vi "Convert Spreadsheet Text to Table.vi"(1 "NumCols":i32=19, 2 "Text In":string="Date: \t8/30/2005\r\nTime: \t7:47 PM\r\nFilename: \tC:\\ER2005\\Data\\Cell 6A Data.dat\r\nProject: \tCell 6A Project\r\nSample ID: \tSample 6A\r\nRock Type: \tRock 6A\r\nFluid Pair: \tmud and guts\r\nRW: \t2.000\r\nRW Temp: \t22.0\r\nFrequency: \t1000\r\nAmplitude: \t1\r\nDAQ Period (mins): \t15\r\nLength: \t10.0000\r\nDiameter: \t5.0000\r\nPorosity: \t33.00\r\nPermeability: \t6.00\r\nElect Spacing: \t5.00\r\n\r\n Point\t Point\t Point\tEl-Time\t ER 1-2\t ER 1-3\t ER 1-4\t ER 2-3\t F 2-3\t Temp-A\t Temp-B\t  NOP\t   Pc\t P-Vol\t  C14\t  C23\r\n  Flag\t  Date\t  Time\t(Hours)\t(ohm-m)\t(ohm-m)\t(ohm-m)\t(ohm-m)\t  ()  \t(deg-C)\t(deg-C)\t (psig)\t (psig)\t  (ml)\t  (pf)\t  (pf)\r\n-------\t-------\t-------\t-------\t-------\t-------\t-------\t-------\t-------\t-------\t-------\t-------\t-------\t-------\t-------\t-------\r\n       \t8/30/05\t 19:47\t   0.00\t 78.495\t 26.215\t 19.742\t  0.075\t    0.8\t  944.1\t  944.0\t    -13\t 113.87\t   0.00\t   9170\t-1836892\r\n   V   \t8/30/05\t 19:55\t   0.14\t 78.256\t 26.179\t 19.715\t  0.178\t    2.0\t  944.0\t  943.9\t      3\t 114.10\t   1.00\t   8175\t-15739120\r\n       \t8/30/05\t 20:01\t   0.23\t 79.415\t 26.786\t 20.250\t  0.472\t    5.2\t  944.0\t  943.9\t      9\t 114.19\t   1.00\t   8342\t 859846\r\n       \t8/30/05\t 20:15\t   0.48\t 79.679\t 26.786\t 20.200\t  0.348\t    3.9\t  944.2\t  944.1\t     -0\t 114.17\t   1.00\t   7967\t-1701240\r\n       \t8/30/05\t 20:30\t   0.73\t 78.752\t 26.296\t 19.774\t  0.073\t    0.8\t  944.7\t  944.6\t      0\t 114.30\t   1.00\t  13499\t-15913632\r\n       \t8/30/05\t 20:45\t   0.98\t 78.717\t 26.274\t 19.757\t  0.053\t    0.6\t  945.4\t  945.3\t     -1\t 114.40\t   1.00\t   7499\t-4510277\r\n       \t8/30/05\t 21:00\t   1.23\t 78.693\t 26.265\t 19.739\t  0.059\t    0.7\t  946.0\t  946.0\t     -4\t 114.44\t   1.00\t   6891\t-35104476\r\n       \t8/30/05\t 21:45\t   1.98\t 78.646\t 26.296\t 19.787\t  0.122\t    1.4\t  946.9\t  946.8\t     -1\t 114.63\t   1.00\t  10271\t3895880\r\n       \t8/30/05\t 22:00\t   2.23\t 78.773\t 26.317\t 19.792\t  0.117\t    1.3\t  947.0\t  946.9\t      2\t 114.68\t   1.00\t   7326\t-26200800\r\n       \t8/30/05\t 22:15\t   2.48\t 78.537\t 26.199\t 19.678\t  0.078\t    0.9\t  947.1\t  947.0\t     -4\t 114.60\t   1.00\t   6067\t-94763630\r\n       \t8/30/05\t 22:30\t   2.73\t 78.642\t 26.240\t 19.708\t  0.090\t    1.0\t  947.1\t  947.0\t      1\t 114.65\t   1.00\t   9512\t-69234673\r\n       \t8/30/05\t 22:45\t   2.98\t 78.652\t 26.227\t 19.714\t  0.014\t    0.2\t  947.1\t  947.0\t     -4\t 114.62\t   1.00\t  14912\t53204022\r\n       \t8/30/05\t 23:00\t   3.23\t 78.582\t 26.218\t 19.703\t  0.041\t    0.5\t  947.1\t  947.0\t     -2\t 114.61\t   1.00\t  11239\t72768719\r\n       \t8/30/05\t 23:30\t   3.73\t 78.459\t 26.247\t 19.741\t  0.167\t    1.9\t  947.1\t  947.0\t    -15\t 114.40\t   1.00\t   8726\t18480066\r\n       \t8/30/05\t 23:45\t   3.98\t 78.835\t 26.447\t 20.018\t  0.275\t    3.1\t  947.0\t  946.9\t     -2\t 114.54\t   1.00\t  14136\t-4576243\r\n       \t8/31/05\t 00:00\t   4.23\t 78.781\t 26.326\t 19.809\t  0.106\t    1.2\t  946.9\t  946.8\t      1\t 114.55\t   1.00\t   8822\t-11848964\r\n       \t8/31/05\t 00:15\t   4.48\t 78.641\t 26.836\t 20.722\t  0.977\t   10.9\t  947.0\t  946.8\t     -7\t 114.44\t   1.00\t   8792\t-1000524\r\n       \t8/31/05\t 00:30\t   4.73\t 78.507\t 26.197\t 19.691\t  0.042\t    0.5\t  946.9\t  946.8\t     -6\t 114.40\t   1.00\t   6399\t4455363\r\n       \t8/31/05\t 00:45\t   4.98\t 78.721\t 26.277\t 19.748\t  0.056\t    0.6\t  946.8\t  946.7\t     -7\t 114.34\t   1.00\t   7223\t3117519\r\n       \t8/31/05\t 01:00\t   5.23\t 78.600\t 27.176\t 21.217\t  1.501\t   16.7\t  946.7\t  946.6\t      1\t 114.41\t   1.00\t   7887\t-430532\r\n       \t8/31/05\t 01:15\t   5.48\t 78.528\t 26.353\t 19.892\t  0.273\t    3.0\t  946.7\t  946.5\t     -5\t 114.27\t   1.00\t   9634\t-2318326\r\n       \t8/31/05\t 01:30\t   5.73\t 78.667\t 26.918\t 20.824\t  1.076\t   12.0\t  946.5\t  946.4\t     -3\t 114.26\t   1.00\t   3410\t-882051\r\n       \t8/31/05\t 01:45\t   5.98\t 78.668\t 26.804\t 20.618\t  0.909\t   10.1\t  946.4\t  946.3\t     -5\t 114.19\t   1.00\t   8867\t-978980\r\n       \t8/31/05\t 02:00\t   6.23\t 78.861\t 27.126\t 21.077\t  1.305\t   14.5\t  946.3\t  946.2\t     -7\t 114.13\t   1.00\t   8074\t-650813\r\n       \t8/31/05\t 02:15\t   6.48\t 78.919\t 27.740\t 22.044\t  2.225\t   24.7\t  946.3\t  946.2\t     -7\t 114.10\t   1.00\t  11911\t-278429\r\n       \t8/31/05\t 02:30\t   6.73\t 78.631\t 29.533\t 24.785\t  5.065\t   56.3\t  946.3\t  946.2\t     -7\t 114.07\t   1.00\t   3196\t-134329\r\n       \t8/31/05\t 02:45\t   6.98\t 78.763\t 28.617\t 23.489\t  3.652\t   40.6\t  946.2\t  946.1\t     -8\t 114.03\t   1.00\t  10850\t-158876\r\n       \t8/31/05\t 03:00\t   7.23\t 78.515\t 28.029\t 22.627\t  2.868\t   31.9\t  946.2\t  946.1\t     -1\t 114.08\t   1.00\t   8849\t-231527\r\n       \t8/31/05\t 03:15\t   7.48\t 78.624\t 28.040\t 22.615\t  2.823\t   31.4\t  946.1\t  946.0\t     -4\t 114.00\t   1.00\t   5831\t-274912\r\n       \t8/31/05\t 03:30\t   7.73\t 78.756\t 27.354\t 21.475\t  1.706\t   19.0\t  946.0\t  945.9\t     -7\t 113.91\t   1.00\t   8002\t-453335\r\n       \t8/31/05\t 03:45\t   7.98\t 78.747\t 26.595\t 20.251\t  0.537\t    6.0\t  946.0\t  945.8\t     -2\t 113.92\t   1.00\t   8616\t-1547600\r\n       \t8/31/05\t 04:00\t   8.23\t 78.815\t 26.629\t 20.295\t  0.558\t    6.2\t  945.9\t  945.8\t     -8\t 113.84\t   1.00\t  12832\t-1325532\r\n       \t8/31/05\t 04:15\t   8.48\t 78.726\t 26.635\t 20.324\t  0.606\t    6.7\t  945.8\t  945.7\t     -2\t 113.86\t   1.00\t   8437\t-1125497\r\n       \t8/31/05\t 04:30\t   8.73\t 78.778\t 27.910\t 22.277\t  2.541\t   28.3\t  945.8\t  945.7\t     -7\t 113.78\t   1.00\t   7602\t-268366\r\n       \t8/31/05\t 04:45\t   8.98\t 78.637\t 26.353\t 19.874\t  0.216\t    2.4\t  945.7\t  945.6\t     -3\t 113.78\t   1.00\t  10193\t-2416454\r\n       \t8/31/05\t 05:00\t   9.23\t 78.599\t 26.390\t 19.850\t  0.290\t    3.2\t  945.6\t  945.5\t     -5\t 113.71\t   1.00\t   5098\t-2269003\r\n       \t8/31/05\t 05:15\t   9.48\t 78.760\t 26.315\t 19.790\t  0.095\t    1.1\t  945.5\t  945.4\t     -3\t 113.67\t   1.00\t   8993\t-4724999\r\n       \t8/31/05\t 05:30\t   9.73\t 78.721\t 26.318\t 19.813\t  0.118\t    1.3\t  945.4\t  945.3\t     -2\t 113.62\t   1.00\t  14097\t-880735\r\n       \t8/31/05\t 05:45\t   9.98\t 78.677\t 26.285\t 19.775\t  0.091\t    1.0\t  945.3\t  945.2\t     -2\t 113.59\t   1.00\t  10441\t-5770254\r\n       \t8/31/05\t 06:00\t  10.23\t 78.754\t 26.289\t 19.828\t  0.081\t    0.9\t  945.2\t  945.1\t     -1\t 113.55\t   1.00\t   8706\t-43779430\r\n       \t8/31/05\t 06:15\t  10.48\t 78.467\t 26.215\t 19.774\t  0.152\t    1.7\t  945.1\t  945.0\t     -4\t 113.48\t   1.00\t  13499\t-28928498\r\n       \t8/31/05\t 06:30\t  10.73\t 78.159\t 26.131\t 19.684\t  0.119\t    1.3\t  945.1\t  945.0\t    -13\t 113.34\t   1.00\t   9406\t10069452\r\n       \t8/31/05\t 06:45\t  10.98\t 78.644\t 26.226\t 19.715\t  0.060\t    0.7\t  945.0\t  944.9\t     -5\t 113.40\t   1.00\t   9232\t-147514498\r\n       \t8/31/05\t 07:00\t  11.23\t 78.685\t 26.235\t 19.715\t  0.041\t    0.5\t  944.9\t  944.8\t     -0\t 113.42\t   1.00\t   9121\t-242772068\r\n       \t8/31/05\t 07:15\t  11.48\t 78.673\t 26.232\t 19.715\t  0.024\t    0.3\t  944.8\t  944.7\t      0\t 113.37\t   1.00\t   9121\t-251192730\r\n       \t8/31/05\t 07:30\t  11.73\t 78.641\t 26.219\t 19.710\t  0.097\t    1.1\t  944.7\t  944.6\t      0\t 113.32\t   1.00\t   9066\t-174139178\r\n       \t8/31/05\t 07:45\t  11.98\t 78.716\t 26.254\t 19.726\t  0.027\t    0.3\t  944.6\t  944.5\t     -1\t 113.26\t   1.00\t   9118\t-67141802\r\n       \t8/31/05\t 08:30\t  12.73\t 78.656\t 26.241\t 19.721\t  0.037\t    0.4\t  944.4\t  944.3\t     -5\t 113.12\t   1.00\t   7506\t-49980234\r\n       \t8/31/05\t 08:45\t  12.98\t 78.651\t 26.273\t 19.754\t  0.087\t    1.0\t  944.3\t  944.2\t      0\t 113.14\t   1.00\t   8945\t-9910310\r\n       \t8/31/05\t 09:00\t  13.23\t 78.651\t 26.244\t 19.730\t  0.042\t    0.5\t  944.2\t  944.1\t     -3\t 113.08\t   1.00\t   9062\t-17571284\r\n       \t8/31/05\t 09:15\t  13.48\t 78.588\t 26.197\t 19.769\t  0.411\t    4.6\t  944.2\t  944.1\t      0\t 113.08\t   1.00\t   4442\t-176818633\r\n       \t8/31/05\t 09:30\t  13.73\t 78.731\t 26.269\t 19.765\t  0.043\t    0.5\t  944.2\t  944.1\t     -2\t 113.05\t   1.00\t   9943\t-42888690\r\n       \t8/31/05\t 09:45\t  13.98\t 78.766\t 26.283\t 19.763\t  0.046\t    0.5\t  944.2\t  944.1\t     -3\t 113.05\t   1.00\t  15116\t-32966750\r\n       \t8/31/05\t 10:00\t  14.23\t 78.774\t 26.280\t 19.754\t  0.068\t    0.8\t  944.3\t  944.2\t     -2\t 113.08\t   1.00\t  14229\t-77196308\r\n       \t8/31/05\t 10:15\t  14.48\t 78.638\t 26.238\t 19.722\t  0.050\t    0.6\t  944.3\t  944.2\t     -4\t 113.10\t   1.00\t   9119\t-60804568\r\n       \t8/31/05\t 10:30\t  14.73\t 78.754\t 26.259\t 19.726\t  0.026\t    0.3\t  944.4\t  944.3\t     -1\t 113.15\t   1.00\t  11845\t-238988649\r\n       \t8/31/05\t 10:45\t  14.98\t 78.473\t 26.200\t 19.731\t  0.063\t    0.7\t  944.6\t  944.5\t    -11\t 113.06\t   1.00\t  11287\t7380698\r\n       \t8/31/05\t 11:00\t  15.23\t 78.616\t 26.238\t 19.726\t  0.054\t    0.6\t  944.6\t  944.5\t     -4\t 113.06\t   1.00\t   8951\t-26403382\r\n       \t8/31/05\t 11:15\t  15.48\t 78.183\t 26.109\t 19.660\t  0.081\t    0.9\t  944.5\t  944.4\t      6\t 113.15\t   1.00\t   4956\t28535656\r\n       \t8/31/05\t 15:21\t  19.58\t 78.281\t 26.162\t 19.728\t  0.196\t    2.2\t  946.2\t  946.1\t    -11\t 113.74\t   1.00\t   7116\t33236548\r\n       \t8/31/05\t 15:37\t  19.84\t 78.610\t 57.318\t 70.043\t 47.045\t  523.2\t  946.1\t  946.0\t      0\t  -0.01\t   1.00\t  11801\t  26360\r\n       \t8/31/05\t 15:51\t  20.08\t 78.088\t 57.173\t 70.177\t 46.970\t  522.4\t  946.3\t  946.2\t      0\t  -0.01\t   1.00\t  13194\t  29551\r\n       \t8/31/05\t 16:10\t  20.40\t 77.565\t 57.005\t 70.339\t 46.860\t  521.4\t  946.6\t  946.5\t      4\t   0.65\t   1.00\t  14980\t  33633\r\n       \t8/31/05\t 17:12\t  21.42\t 78.472\t 57.260\t 70.009\t 47.015\t  523.3\t  946.9\t  946.8\t     12\t   0.06\t   1.00\t  11981\t  26818\r\n       \t8/31/05\t 18:30\t  22.73\t 79.980\t 57.628\t 69.742\t 47.128\t   26.9\t   28.0\t   28.2\t      0\t  -0.02\t   1.00\t   9052\t  20081\r\n       \t8/31/05\t 18:45\t  22.98\t 78.373\t 57.216\t 69.974\t 46.991\t   26.9\t   28.0\t   28.2\t     -1\t   0.00\t   1.00\t  12054\t  26951\r\n       \t8/31/05\t 19:00\t  23.23\t 77.553\t 56.964\t 70.267\t 46.812\t   26.8\t   28.0\t   28.2\t     -1\t  -0.01\t   1.00\t  14876\t  33415\r\n       \t8/31/05\t 19:15\t  23.48\t 78.551\t 57.273\t 69.999\t 47.003\t   26.9\t   28.1\t   28.3\t      0\t   0.00\t   1.00\t  11874\t  26549\r\n       \t8/31/05\t 19:30\t  23.73\t 78.556\t 57.291\t 70.038\t 47.021\t   26.9\t   28.1\t   28.4\t      0\t  -0.01\t   1.00\t  11945\t  26713\r\n       \t8/31/05\t 19:45\t  23.98\t 78.462\t 57.249\t 70.019\t 46.992\t   26.9\t   28.1\t   28.3\t      0\t  -0.01\t   1.00\t  12089\t  27040\r\n       \t8/31/05\t 20:00\t  24.23\t 78.408\t 57.215\t 69.974\t 46.972\t   26.9\t   28.1\t   28.3\t     -0\t  -0.02\t   1.00\t  12054\t  26981\r\n       \t8/31/05\t 20:15\t  24.48\t 78.477\t 57.253\t 70.016\t 46.994\t   27.0\t   28.2\t   28.4\t      0\t  -0.01\t   1.00\t  12053\t  26958\r\n       \t8/31/05\t 20:30\t  24.73\t 78.428\t 57.236\t 70.010\t 46.992\t   27.0\t   28.3\t   28.4\t      0\t  -0.01\t   1.00\t  12089\t  27063\r\n       \t8/31/05\t 20:45\t  24.98\t 78.428\t 57.238\t 70.010\t 46.992\t   27.0\t   28.3\t   28.4\t      0\t  -0.01\t   1.00\t  12089\t  27037\r\n       \t8/31/05\t 21:00\t  25.23\t 78.428\t 57.236\t 70.010\t 46.992\t   26.9\t   28.2\t   28.4\t     -4\t   0.04\t   1.00\t  12089\t  27063\r\n       \t8/31/05\t 21:15\t  25.48\t 78.536\t 57.283\t 70.026\t 47.023\t   26.9\t   28.2\t   28.4\t     -1\t  -0.00\t   1.00\t  11909\t  26628\r\n       \t8/31/05\t 21:30\t  25.73\t 78.556\t 57.302\t 70.038\t 47.039\t   27.0\t   28.2\t   28.5\t      0\t  -0.02\t   1.00\t  11945\t  26717\r\n       \t8/31/05\t 21:45\t  25.98\t 78.482\t 57.271\t 70.055\t 47.012\t   26.9\t   28.1\t   28.3\t      0\t  -0.01\t   1.00\t  12123\t  27122\r\n       \t8/31/05\t 22:00\t  26.23\t 78.452\t 57.227\t 69.965\t 46.978\t   26.9\t   28.2\t   28.3\t      1\t  -0.01\t   1.00\t  11947\t  26736\r\n       \t8/31/05\t 22:15\t  26.48\t 79.896\t 57.649\t 69.863\t 47.159\t   27.0\t   28.1\t   28.3\t      0\t  -0.02\t   1.00\t   9407\t  20928\r\n       \t8/31/05\t 22:30\t  26.73\t 78.126\t 57.155\t 70.085\t 46.949\t   26.8\t   28.1\t   28.2\t     -0\t  -0.02\t   1.00\t  12875\t  28813\r\n       \t8/31/05\t 22:45\t  26.98\t 79.049\t 57.429\t 69.939\t 47.095\t   26.9\t   28.0\t   28.2\t      0\t  -0.02\t   1.00\t  10801\t  24092\r\n       \t8/31/05\t 23:00\t  27.23\t 79.738\t 57.586\t 69.804\t 47.131\t   26.9\t   28.0\t   28.1\t     -0\t  -0.01\t   1.00\t   9480\t  21041\r\n       \t8/31/05\t 23:15\t  27.48\t 78.149\t 57.190\t 70.130\t 46.986\t   26.8\t   27.9\t   28.1\t      1\t  -0.02\t   1.00\t  12909\t  28869\r\n       \t8/31/05\t 23:30\t  27.73\t 78.421\t 57.249\t 70.019\t 47.009\t   26.7\t   27.8\t   28.0\t      0\t  -0.02\t   1.00\t  12089\t  26987\r\n       \t8/31/05\t 23:45\t  27.98\t 78.517\t 57.272\t 69.999\t 47.021\t   26.7\t   27.7\t   27.9\t     -0\t  -0.02\t   1.00\t  11874\t  26573\r\n       \t9/1/05\t 00:00\t  28.23\t 78.442\t 57.252\t 70.016\t 47.011\t   26.6\t   27.6\t   27.8\t      0\t  -0.03\t   1.00\t  12053\t  26982\r\n       \t9/1/05\t 00:15\t  28.48\t 77.527\t 56.980\t 70.346\t 46.829\t   26.5\t   27.5\t   27.7\t      0\t  -0.03\t   1.00\t  15195\t  34126\r\n       \t9/1/05\t 00:30\t  28.73\t 78.700\t 57.351\t 70.009\t 47.077\t   26.6\t   27.5\t   27.6\t     -0\t  -0.02\t   1.00\t  11516\t  25706\r\n       \t9/1/05\t 00:45\t  28.98\t 78.491\t 57.286\t 70.060\t 47.030\t   26.5\t   27.4\t   27.6\t     -0\t  -0.04\t   1.00\t  12087\t  27018\r\n       \t9/1/05\t 01:00\t  29.23\t 78.042\t 57.154\t 70.128\t 46.971\t   26.5\t   27.3\t   27.5\t      0\t  -0.04\t   1.00\t  13124\t  29385\r\n       \t9/1/05\t 01:15\t  29.48\t 79.870\t 57.630\t 69.798\t 47.158\t   26.5\t   27.3\t   27.4\t      0\t  -0.03\t   1.00\t   9265\t  20552\r\n       \t9/1/05\t 01:30\t  29.73\t 78.436\t 57.264\t 70.025\t 47.028\t   26.4\t   27.2\t   27.3\t      0\t  -0.03\t   1.00\t  12053\t  26933\r\n       \t9/1/05\t 01:45\t  29.98\t 78.545\t 57.308\t 70.041\t 47.058\t   26.4\t   27.1\t   27.3\t      0\t  -0.04\t   1.00\t  11873\t  26551\r\n       \t9/1/05\t 02:00\t  30.23\t 78.779\t 57.327\t 69.916\t 47.032\t   26.3\t   27.0\t   27.2\t      0\t  -0.03\t   1.00\t  11196\t  24965\r\n       \t9/1/05\t 02:15\t  30.48\t 78.019\t 57.147\t 70.136\t 46.967\t   26.2\t   27.0\t   27.1\t      0\t  -0.04\t   1.00\t  13196\t  29549\r\n       \t9/1/05\t 02:30\t  30.73\t 78.480\t 57.264\t 70.015\t 47.016\t   26.2\t   26.9\t   27.0\t     -0\t  -0.04\t   1.00\t  11945\t  26684\r\n       \t9/1/05\t 02:45\t  30.98\t 78.451\t 57.255\t 70.022\t 47.012\t   26.2\t   26.8\t   27.0\t      0\t  -0.04\t   1.00\t  12017\t  26874\r\n       \t9/1/05\t 03:00\t  31.23\t 78.534\t 57.297\t 70.060\t 47.035\t   26.2\t   26.7\t   26.9\t      0\t  -0.03\t   1.00\t  11980\t  26770\r\n       \t9/1/05\t 03:15\t  31.48\t 78.436\t 57.264\t 70.034\t 47.028\t   26.1\t   26.6\t   26.8\t      1\t  -0.04\t   1.00\t  12052\t  26930\r\n       \t9/1/05\t 03:30\t  31.73\t 77.578\t 57.010\t 70.331\t 46.865\t   25.9\t   26.5\t   26.7\t      0\t  -0.04\t   1.00\t  14909\t  33469\r\n       \t9/1/05\t 03:45\t  31.98\t 78.535\t 57.309\t 70.069\t 47.053\t   26.0\t   26.4\t   26.6\t      1\t  -0.04\t   1.00\t  11979\t  26770\r\n       \t9/1/05\t 04:00\t  32.23\t 78.491\t 57.262\t 69.982\t 47.018\t   25.9\t   26.4\t   26.5\t     -0\t  -0.05\t   1.00\t  11839\t  26439\r\n       \t9/1/05\t 04:15\t  32.48\t 78.436\t 57.264\t 70.034\t 47.028\t   25.9\t   26.3\t   26.4\t      1\t  -0.05\t   1.00\t  12052\t  26930\r\n       \t9/1/05\t 04:30\t  32.73\t 79.166\t 57.475\t 69.951\t 47.120\t   25.9\t   26.2\t   26.3\t      1\t  -0.06\t   1.00\t  10622\t  23661\r\n       \t9/1/05\t 04:45\t  32.98\t 78.918\t 57.408\t 69.987\t 47.100\t   25.8\t   26.1\t   26.2\t      0\t  -0.05\t   1.00\t  11050\t  24637\r\n       \t9/1/05\t 05:00\t  33.23\t 78.186\t 57.223\t 70.147\t 47.028\t   25.8\t   26.1\t   26.1\t      1\t  -0.05\t   1.00\t  12801\t  28647\r\n       \t9/1/05\t 05:15\t  33.48\t 78.451\t 57.279\t 70.040\t 47.048\t   25.7\t   25.9\t   26.1\t      1\t  -0.06\t   1.00\t  12016\t  26849\r\n       \t9/1/05\t 05:30\t  33.73\t 78.451\t 57.278\t 70.040\t 47.048\t   25.7\t   25.9\t   26.0\t      1\t  -0.05\t   1.00\t  12016\t  26875\r\n       \t9/1/05\t 05:45\t  33.98\t 78.520\t 57.316\t 70.081\t 47.069\t   25.7\t   25.9\t   25.9\t      0\t  -0.05\t   1.00\t  12015\t  26879\r\n       \t9/1/05\t 06:00\t  34.23\t 78.451\t 57.278\t 70.040\t 47.048\t   25.6\t   25.7\t   25.9\t      1\t  -0.05\t   1.00\t  12016\t  26875\r\n       \t9/1/05\t 06:15\t  34.48\t 78.579\t 57.321\t 70.068\t 47.059\t   25.6\t   25.6\t   25.8\t      0\t  -0.05\t   1.00\t  11872\t  26522\r\n       \t9/1/05\t 06:30\t  34.73\t 78.449\t 57.282\t 70.055\t 47.043\t   25.5\t   25.5\t   25.7\t      0\t  -0.05\t   1.00\t  12087\t  26992\r\n       \t9/1/05\t 06:45\t  34.98\t 78.520\t 57.305\t 70.081\t 47.052\t   25.5\t   25.4\t   25.6\t     -0\t  -0.05\t   1.00\t  12015\t  26849\r\n       \t9/1/05\t 07:00\t  35.23\t 78.456\t 57.270\t 70.055\t 47.026\t   25.4\t   25.4\t   25.5\t      1\t  -0.06\t   1.00\t  12087\t  27039\r\n       \t9/1/05\t 07:15\t  35.48\t 78.558\t 57.328\t 70.080\t 47.073\t   25.4\t   25.2\t   25.4\t      0\t  -0.04\t   1.00\t  11907\t  26581\r\n       \t9/1/05\t 07:30\t  35.73\t 78.499\t 57.312\t 70.093\t 47.066\t   25.3\t   25.2\t   25.3\t      2\t  -0.04\t   1.00\t  12050\t  26908\r\n       \t9/1/05\t 07:45\t  35.98\t 78.499\t 57.312\t 70.093\t 47.066\t   25.3\t   25.0\t   25.2\t      1\t  -0.04\t   1.00\t  12050\t  26908\r\n       \t9/1/05\t 08:00\t  36.23\t 78.456\t 57.282\t 70.064\t 47.044\t   25.2\t   24.9\t   25.1\t      0\t  -0.05\t   1.00\t  12087\t  27039\r\n       \t9/1/05\t 08:15\t  36.48\t 78.849\t 57.374\t 69.943\t 47.071\t   25.2\t   24.9\t   25.0\t      1\t  -0.05\t   1.00\t  11088\t  24649\r\n       \t9/1/05\t 08:30\t  36.73\t 78.415\t 57.282\t 70.064\t 47.061\t   25.1\t   24.8\t   25.0\t      2\t  -0.04\t   1.00\t  12087\t  26987\r\n       \t9/1/05\t 08:45\t  36.98\t 79.221\t 57.493\t 69.917\t 47.145\t   25.2\t   24.8\t   24.9\t      1\t  -0.04\t   1.00\t  10372\t  23061\r\n       \t9/1/05\t 09:00\t  37.23\t 79.177\t 57.490\t 69.975\t 47.138\t   25.1\t   24.7\t   24.8\t      1\t  -0.06\t   1.00\t  10585\t  23551\r\n       \t9/1/05\t 09:15\t  37.48\t 78.484\t 57.320\t 70.106\t 47.082\t   25.1\t   24.7\t   24.8\t      1\t  -0.06\t   1.00\t  12085\t  26990\r\n       \t9/1/05\t 09:30\t  37.73\t 78.493\t 57.306\t 70.064\t 47.066\t   25.1\t   24.7\t   24.9\t      1\t  -0.05\t   1.00\t  11979\t  26745\r\n       \t9/1/05\t 09:45\t  37.98\t 77.556\t 57.026\t 70.370\t 46.892\t   25.0\t   24.8\t   24.9\t      2\t  -0.04\t   1.00\t  15015\t  33660\r\n       \t9/1/05\t 10:00\t  38.23\t 78.459\t 57.294\t 70.055\t 47.066\t   25.1\t   24.8\t   24.9\t      2\t  -0.04\t   1.00\t  11980\t  26741\r\n       \t9/1/05\t 10:15\t  38.48\t 78.430\t 57.285\t 70.061\t 47.062\t   25.2\t   24.9\t   25.0\t      1\t  -0.05\t   1.00\t  12051\t  26931\r\n       \t9/1/05\t 10:30\t  38.73\t 78.450\t 57.281\t 70.064\t 47.042\t   25.2\t   25.0\t   25.1\t      1\t  -0.04\t   1.00\t  12087\t  27016\r\n       \t9/1/05\t 10:45\t  38.98\t 79.143\t 57.490\t 69.966\t 47.156\t   25.3\t   25.0\t   25.2\t      2\t  -0.05\t   1.00\t  10585\t  23552\r\n       \t9/1/05\t 11:00\t  39.23\t 78.202\t 57.230\t 70.169\t 47.024\t   25.2\t   25.1\t   25.2\t      1\t  -0.06\t   1.00\t  12836\t  28707\r\n       \t9/1/05\t 11:15\t  39.48\t 79.396\t 57.526\t 69.883\t 47.141\t   25.3\t   25.1\t   25.2\t      2\t  -0.06\t   1.00\t  10051\t  22324\r\n       \t9/1/05\t 11:30\t  39.73\t 78.543\t 57.324\t 70.084\t 47.072\t   25.3\t   25.1\t   25.3\t      1\t  -0.04\t   1.00\t  11943\t  26663\r\n       \t9/1/05\t 11:45\t  39.98\t 78.484\t 57.308\t 70.097\t 47.064\t   25.4\t   25.2\t   25.4\t      1\t  -0.04\t   1.00\t  12086\t  26990\r\n       \t9/1/05\t 12:00\t  40.23\t 78.430\t 57.274\t 70.052\t 47.045\t   25.3\t   25.2\t   25.4\t      1\t  -0.07\t   1.00\t  12052\t  26904\r\n       \t9/1/05\t 13:18\t  41.53\t 78.459\t 57.282\t 70.036\t 47.048\t   25.7\t   25.8\t   26.1\t      1\t  -0.05\t   1.00\t  11980\t  26744\r\n       \t9/1/05\t 15:36\t  43.82\t 78.712\t 57.321\t 69.929\t 47.043\t   26.3\t   26.9\t   27.2\t      1\t  -0.10\t   1.00\t  11339\t  25297\r\n       \t9/1/05\t 16:35\t  44.81\t 78.487\t 57.276\t 70.015\t 47.035\t   26.6\t   27.5\t   27.7\t      1\t  -0.08\t   1.00\t  11945\t  26737\r\n       \t9/1/05\t 16:50\t  45.06\t 77.738\t 57.050\t 70.232\t 46.892\t   26.5\t   27.5\t   27.7\t     -1\t  -0.09\t   1.00\t  14196\t  31888\r\n       \t9/1/05\t 17:05\t  45.31\t 77.608\t 57.022\t 70.349\t 46.868\t   26.6\t   27.7\t   27.9\t      1\t  -0.11\t   1.00\t  14944\t  33605\r\n       \t9/1/05\t 17:20\t  45.56\t 77.945\t 57.113\t 70.152\t 46.936\t   26.7\t   27.8\t   28.0\t     -1\t  -0.11\t   1.00\t  13446\t  30171\r\n       \t9/1/05\t 17:35\t  45.81\t 78.367\t 57.215\t 69.974\t 46.989\t   26.8\t   27.9\t   28.1\t     -0\t  -0.11\t   1.00\t  12054\t  26928\r\n       \t9/1/05\t 17:50\t  46.06\t 78.472\t 57.248\t 70.000\t 46.997\t   26.9\t   28.0\t   28.2\t      0\t  -0.10\t   1.00\t  11982\t  26818\r\n       \t9/1/05\t 18:05\t  46.31\t 78.059\t 57.152\t 70.170\t 46.947\t   26.9\t   28.1\t   28.3\t     -1\t  -0.09\t   1.00\t  13302\t  29849\r\n       \t9/1/05\t 18:20\t  46.56\t 78.452\t 57.241\t 69.988\t 46.999\t   26.9\t   28.2\t   28.4\t     -1\t  -0.10\t   1.00\t  11946\t  26732\r\n       \t9/1/05\t 18:35\t  46.81\t 78.492\t 57.271\t 70.036\t 47.017\t   27.0\t   28.3\t   28.5\t      1\t  -0.10\t   1.00\t  12016\t  26873\r\n       \t9/1/05\t 18:50\t  47.06\t 78.856\t 57.359\t 69.909\t 47.062\t   27.1\t   28.4\t   28.6\t      0\t  -0.11\t   1.00\t  11053\t  24665\r\n       \t9/1/05\t 19:05\t  47.31\t 78.521\t 57.279\t 70.029\t 47.021\t   27.1\t   28.5\t   28.7\t     -0\t  -0.10\t   1.00\t  11945\t  26710\r\n       \t9/1/05\t 19:20\t  47.56\t 78.497\t 57.275\t 70.042\t 47.014\t   27.1\t   28.5\t   28.7\t     -1\t  -0.11\t   1.00\t  12088\t  27043\r\n       \t9/1/05\t 19:35\t  47.81\t 79.868\t 57.614\t 69.768\t 47.142\t   27.3\t   28.6\t   28.8\t     -1\t  -0.11\t   1.00\t   9230\t  20492\r\n       \t9/1/05\t 19:50\t  48.06\t 78.926\t 57.378\t 69.897\t 47.069\t   27.3\t   28.7\t   28.9\t     -1\t  -0.11\t   1.00\t  10910\t  24337\r\n       \t9/1/05\t 20:05\t  48.31\t 80.015\t 57.642\t 69.756\t 47.132\t   27.3\t   28.8\t   28.9\t     -1\t  -0.11\t   1.00\t   9051\t  20083\r\n       \t9/1/05\t 20:20\t  48.56\t 80.027\t 57.653\t 69.751\t 47.152\t   27.4\t   28.8\t   29.0\t     -0\t  -0.11\t   1.00\t   8980\t  19919\r\n       \t9/1/05\t 20:35\t  48.81\t 78.532\t 57.264\t 69.978\t 47.004\t   27.3\t   28.9\t   29.1\t     -0\t  -0.11\t   1.00\t  11839\t  26493\r\n       \t9/1/05\t 20:50\t  49.06\t 78.487\t 57.253\t 69.988\t 47.000\t   27.3\t   28.9\t   29.1\t      0\t  -0.11\t   1.00\t  11946\t  26712\r\n       \t9/1/05\t 21:05\t  49.31\t 78.247\t 57.188\t 70.045\t 46.968\t   27.3\t   28.9\t   29.1\t     -0\t  -0.10\t   1.00\t  12554\t  28103\r\n       \t9/1/05\t 21:20\t  49.56\t 78.477\t 57.267\t 70.030\t 47.015\t   27.3\t   28.9\t   29.1\t     -0\t  -0.10\t   1.00\t  12052\t  26958\r\n       \t9/1/05\t 21:35\t  49.81\t 78.437\t 57.249\t 69.991\t 47.016\t   27.4\t   29.0\t   29.1\t     -0\t  -0.10\t   1.00\t  11982\t  26791\r\n       \t9/1/05\t 21:50\t  50.06\t 79.013\t 57.408\t 69.926\t 47.074\t   27.4\t   28.9\t   29.1\t     -0\t  -0.10\t   1.00\t  10873\t  24258\r\n       \t9/1/05\t 22:05\t  50.31\t 79.946\t 57.614\t 69.763\t 47.109\t   27.4\t   28.9\t   29.1\t      0\t  -0.10\t   1.00\t   9159\t  20323\r\n       \t9/1/05\t 22:20\t  50.56\t 77.561\t 56.981\t 70.306\t 46.824\t   27.2\t   28.8\t   29.0\t     -0\t  -0.10\t   1.00\t  15018\t  33717\r\n       \t9/1/05\t 22:35\t  50.81\t 77.697\t 57.041\t 70.282\t 46.876\t   27.2\t   28.8\t   28.9\t     -0\t  -0.10\t   1.00\t  14516\t  32600\r\n       \t9/1/05\t 22:50\t  51.06\t 78.526\t 57.283\t 70.036\t 47.017\t   27.3\t   28.8\t   28.9\t     -0\t  -0.11\t   1.00\t  12016\t  26880\r\n       \t9/1/05\t 23:05\t  51.31\t 78.521\t 57.280\t 70.020\t 47.022\t   27.3\t   28.8\t   28.9\t      0\t  -0.10\t   1.00\t  11945\t  26686\r\n       \t9/1/05\t 23:20\t  51.56\t 80.168\t 57.687\t 69.737\t 47.161\t   27.3\t   28.7\t   28.9\t      0\t  -0.09\t   1.00\t   8765\t  19428\r\n       \t9/1/05\t 23:35\t  51.81\t 78.506\t 57.275\t 70.023\t 47.019\t   27.2\t   28.6\t   28.8\t      0\t  -0.11\t   1.00\t  11981\t  26794\r\n       \t9/1/05\t 23:50\t  52.06\t 77.574\t 56.997\t 70.278\t 46.858\t   27.1\t   28.6\t   28.8\t      0\t  -0.10\t   1.00\t  14768\t  33194\r\n       \t9/2/05\t 00:05\t  52.31\t 78.536\t 57.295\t 70.026\t 47.041\t   27.1\t   28.5\t   28.7\t      0\t  -0.11\t   1.00\t  11909\t  26631\r\n       \t9/2/05\t 00:20\t  52.56\t 78.442\t 57.253\t 70.007\t 47.012\t   27.1\t   28.4\t   28.6\t      0\t  -0.10\t   1.00\t  12053\t  26958\r\n       \t9/2/05\t 00:35\t  52.81\t 77.649\t 57.025\t 70.315\t 46.861\t   26.9\t   28.3\t   28.5\t      1\t  -0.10\t   1.00\t  14730\t  33038\r\n       \t9/2/05\t 00:50\t  53.06\t 78.497\t 57.287\t 70.051\t 47.032\t   27.0\t   28.3\t   28.4\t     -0\t  -0.11\t   1.00\t  12087\t  27044\r\n       \t9/2/05\t 01:05\t  53.31\t 80.190\t 57.712\t 69.791\t 47.179\t   27.1\t   28.2\t   28.4\t      0\t  -0.10\t   1.00\t   8836\t  19617\r\n       \t9/2/05\t 01:20\t  53.56\t 78.487\t 57.279\t 70.029\t 47.039\t   26.9\t   28.1\t   28.3\t      0\t  -0.10\t   1.00\t  11945\t  26707\r\n       \t9/2/05\t 01:35\t  53.81\t 79.130\t 57.412\t 69.836\t 47.068\t   26.9\t   28.0\t   28.2\t      1\t  -0.11\t   1.00\t  10446\t  23297\r\n       \t9/2/05\t 01:50\t  54.06\t 79.031\t 57.423\t 69.942\t 47.093\t   26.9\t   27.9\t   28.1\t      1\t  -0.11\t   1.00\t  10837\t  24200\r\n       \t9/2/05\t 02:05\t  54.31\t 79.961\t 57.656\t 69.816\t 47.164\t   26.9\t   27.9\t   28.1\t     -1\t  -0.10\t   1.00\t   9193\t  20435\r\n       \t9/2/05\t 02:20\t  54.56\t 77.565\t 56.994\t 70.321\t 46.843\t   26.6\t   27.8\t   28.0\t      0\t  -0.10\t   1.00\t  14981\t  33609\r\n       \t9/2/05\t 02:35\t  54.81\t 78.487\t 57.264\t 70.006\t 47.017\t   26.7\t   27.7\t   27.9\t      0\t  -0.11\t   1.00\t  11946\t  26737\r\n       \t9/2/05\t 02:50\t  55.06\t 78.436\t 57.252\t 70.016\t 47.010\t   26.7\t   27.7\t   27.8\t      0\t  -0.11\t   1.00\t  12053\t  26932\r\n       \t9/2/05\t 03:05\t  55.31\t 79.759\t 57.592\t 69.802\t 47.132\t   26.7\t   27.6\t   27.8\t      0\t  -0.11\t   1.00\t   9444\t  20959\r\n       \t9/2/05\t 03:20\t  55.56\t 80.166\t 57.712\t 69.805\t 47.176\t   26.7\t   27.6\t   27.8\t      0\t  -0.15\t   1.00\t   8907\t  19734\r\n       \t9/2/05\t 03:35\t  55.81\t 78.456\t 57.260\t 70.028\t 47.009\t   26.6\t   27.4\t   27.6\t      0\t  -0.11\t   1.00\t  12088\t  27017\r\n       \t9/2/05\t 03:50\t  56.06\t 78.480\t 57.274\t 70.015\t 47.033\t   26.5\t   27.4\t   27.6\t      1\t  -0.11\t   1.00\t  11945\t  26714\r\n       \t9/2/05\t 04:05\t  56.31\t 78.451\t 57.268\t 70.022\t 47.030\t   26.5\t   27.3\t   27.5\t      0\t  -0.11\t   1.00\t  12017\t  26851\r\n       \t9/2/05\t 04:20\t  56.56\t 78.515\t 57.301\t 70.047\t 47.055\t   26.4\t   27.2\t   27.4\t      0\t  -0.10\t   1.00\t  11944\t  26688\r\n       \t9/2/05\t 04:35\t  56.81\t 78.421\t 57.260\t 70.028\t 47.027\t   26.4\t   27.1\t   27.3\t      0\t  -0.12\t   1.00\t  12088\t  27014\r\n       \t9/2/05\t 04:50\t  57.06\t 78.485\t 57.293\t 70.054\t 47.052\t   26.4\t   27.1\t   27.3\t      0\t  -0.11\t   1.00\t  12016\t  26851\r\n       \t9/2/05\t 05:05\t  57.31\t 78.456\t 57.286\t 70.060\t 47.048\t   26.3\t   27.0\t   27.2\t      0\t  -0.11\t   1.00\t  12087\t  27015\r\n       \t9/2/05\t 05:20\t  57.56\t 79.058\t 57.430\t 69.922\t 47.092\t   26.3\t   26.9\t   27.1\t      1\t  -0.11\t   1.00\t  10766\t  23991\r\n       \t9/2/05\t 05:35\t  57.81\t 77.686\t 57.061\t 70.322\t 46.908\t   26.2\t   26.9\t   27.1\t      0\t  -0.09\t   1.00\t  14550\t  32653\r\n       \t9/2/05\t 05:50\t  58.06\t 78.505\t 57.289\t 70.066\t 47.032\t   26.2\t   26.8\t   27.0\t      1\t  -0.12\t   1.00\t  12051\t  26933\r\n       \t9/2/05\t 06:05\t  58.31\t 78.470\t 57.264\t 70.034\t 47.010\t   26.2\t   26.8\t   27.0\t      1\t  -0.11\t   1.00\t  12052\t  26933\r\n       \t9/2/05\t 06:20\t  58.56\t 78.560\t 57.288\t 70.014\t 47.021\t   26.2\t   26.8\t   26.9\t      0\t  -0.11\t   1.00\t  11838\t  26442\r\n       \t9/2/05\t 06:35\t  58.81\t 77.957\t 57.135\t 70.221\t 46.945\t   26.1\t   26.7\t   26.9\t      1\t  -0.11\t   1.00\t  13622\t  30532\r\n       \t9/2/05\t 06:50\t  59.06\t 77.974\t 57.133\t 70.159\t 46.958\t   26.1\t   26.7\t   26.8\t      0\t  -0.09\t   1.00\t  13338\t  29900\r\n       \t9/2/05\t 07:05\t  59.31\t 78.465\t 57.272\t 70.027\t 47.032\t   26.1\t   26.7\t   26.8\t      0\t  -0.09\t   1.00\t  11981\t  26766\r\n       \t9/2/05\t 07:20\t  59.56\t 78.387\t 57.234\t 70.005\t 47.005\t   26.0\t   26.6\t   26.7\t      2\t  -0.11\t   1.00\t  12089\t  27011\r\n       \t9/2/05\t 07:35\t  59.81\t 78.549\t 57.313\t 70.065\t 47.055\t   26.1\t   26.6\t   26.7\t      1\t  -0.12\t   1.00\t  11944\t  26688\r\n       \t9/2/05\t 07:50\t  60.06\t 78.480\t 57.276\t 70.024\t 47.034\t   26.1\t   26.6\t   26.7\t      0\t  -0.10\t   1.00\t  11945\t  26684\r\n       \t9/2/05\t 08:05\t  60.31\t 79.480\t 57.537\t 69.868\t 47.127\t   26.1\t   26.5\t   26.7\t      1\t  -0.11\t   1.00\t   9979\t  22188\r\n       \t9/2/05\t 08:20\t  60.56\t 78.405\t 57.274\t 70.099\t 47.037\t   25.9\t   26.4\t   26.5\t      0\t  -0.10\t   1.00\t  12301\t  27506\r\n       \t9/2/05\t 08:35\t  60.81\t 78.505\t 57.300\t 70.075\t 47.049\t   26.0\t   26.5\t   26.5\t      1\t  -0.12\t   1.00\t  12051\t  26960\r\n       \t9/2/05\t 08:50\t  61.06\t 79.972\t 57.668\t 69.803\t 47.182\t   25.9\t   26.2\t   26.3\t      2\t  -0.10\t   1.00\t   9086\t  20118\r\n       \t9/2/05\t 09:05\t  61.31\t 78.465\t 57.282\t 70.036\t 47.050\t   25.7\t   26.0\t   26.0\t      0\t  -0.10\t   1.00\t  11980\t  26793\r\n       \t9/2/05\t 09:20\t  61.56\t 78.480\t 57.275\t 70.033\t 47.033\t   25.8\t   26.2\t   26.3\t      1\t  -0.09\t   1.00\t  11945\t  26708\r\n       \t9/2/05\t 09:36\t  61.83\t 78.223\t 57.253\t 70.148\t 47.008\t   25.9\t   26.3\t   26.5\t      1\t  -0.11\t   1.00\t  12422\t  27164\r\n       \t9/2/05\t 09:50\t  62.06\t 78.320\t 57.212\t 70.004\t 47.005\t   25.9\t   26.4\t   26.5\t      2\t  -0.11\t   1.00\t  12088\t  27055\r\n       \t9/2/05\t 10:05\t  62.31\t 78.644\t 57.226\t 69.865\t 47.012\t   26.0\t   26.5\t   26.6\t      1\t  -0.10\t   1.00\t  11633\t  26656\r\n       \t9/2/05\t 10:20\t  62.56\t 79.006\t 57.246\t 69.746\t 47.011\t   26.1\t   26.6\t   26.8\t      1\t  -0.10\t   1.00\t  11230\t  26297\r\n       \t9/2/05\t 10:35\t  62.81\t 78.457\t 57.223\t 69.945\t 47.008\t   26.2\t   26.9\t   27.0\t      0\t  -0.10\t   1.00\t  11898\t  26835\r\n       \t9/2/05\t 10:50\t  63.06\t 78.739\t 57.242\t 69.858\t 47.008\t   26.2\t   26.9\t   27.0\t      0\t  -0.09\t   1.00\t  11579\t  26618\r\n       \t9/2/05\t 11:06\t  63.33\t 78.403\t 57.241\t 70.016\t 47.005\t   26.3\t   27.0\t   27.2\t      1\t  -0.10\t   1.00\t  12065\t  26943") -> (7 "Table Out":string[][](table))   [LabVIEW 2013]
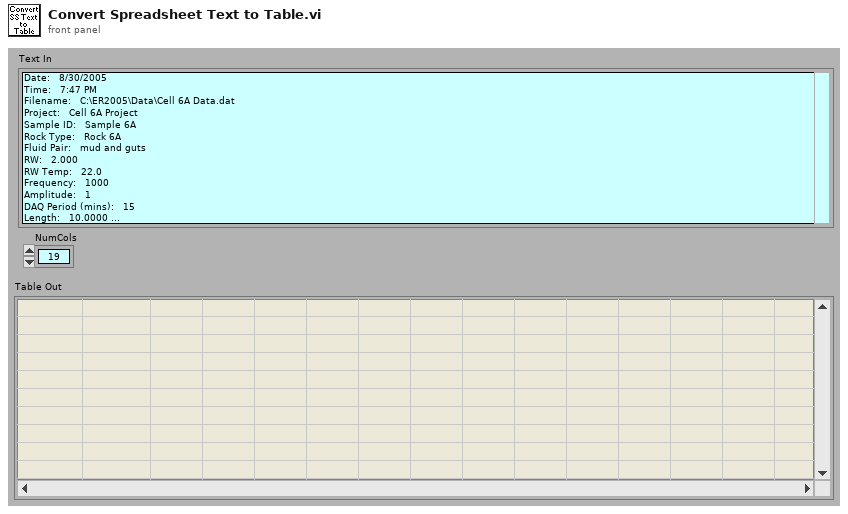
[diagram p1: front panel]
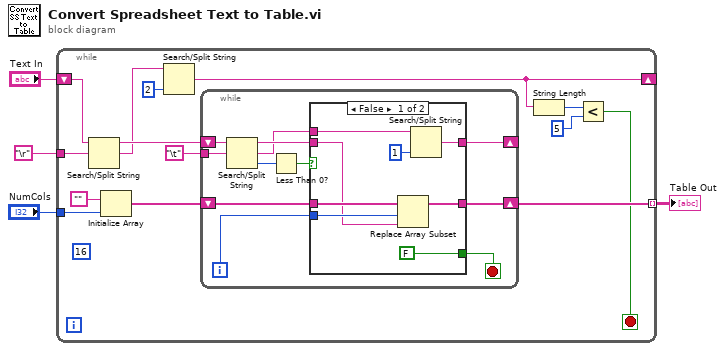
[diagram p0: block diagram]
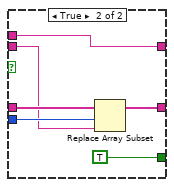
[diagram p2: hidden frame]
diagram:
  n1 = while {
    shift-right: [w9] -> _
    shift-left: "Text In" -> [w18]
    tunnel: "\r" -> [w17]
    tunnel: [w12] -> w2 mode=indexing
    tunnel: "NumCols" -> [w5]
    stop <- w6 stop-if-true
    (unwired) 16 ("dimension size")
    n2 = Search/Split String(string=w18, search string/char (-)=w17) -> (substring before match=w16:string, match + rest of string=w13:string)  [unwired: 1 in, 1 out]
    n3 = Initialize Array("", w5) -> (w14:string[])
    n4 = Search/Split String(string=w13, offset (0)=2) -> (match + rest of string=w9:string)  [unwired: 1 in, 2 out]
    n5 = while {
      shift-right: [w23] -> _
      shift-left: w16 -> [w29]
      tunnel: "\t" -> [w28]
      shift-right: [w19] -> w12
      shift-left: w14 -> [w22]
      i -> [w21]
      stop <- w25 stop-if-true
      n6 = Search/Split String(string=w29, search string/char (-)=w28) -> (substring before match=w24:string, match + rest of string=w20:string, offset of match=w27:i32)  [unwired: 1 in]
      n7 = Less Than 0?(x=w27) -> (x < 0?=w26:bool)
      n8 = case shown="False" w26 {
        tunnel: [FALSE TRUE] -> w25
        tunnel: w24 -> [w32 w39]
        tunnel: [w36 w42] -> w23
        tunnel: w22 -> [w35 w41]
        tunnel: w21 -> [w34 w40]
        tunnel: w20 -> [w33 w42]
        tunnel: [w31 w38] -> w19
        frame False {
          n9 = Replace Array Subset(array=w35, new element=w32, index=w34) -> (w31:string[])
          n10 = Search/Split String(string=w33, offset (0)=1) -> (match + rest of string=w36:string)  [unwired: 1 in, 2 out]
        }
        frame True {
          n11 = Replace Array Subset(array=w41, new element=w39, index=w40) -> (w38:string[])
        }
      }
    }
    n12 = String Length(string=w9) -> (length=w8:i32)
    n13 = Less?(x=w8, y=5) -> (x < y?=w6:bool)
  }
  "Table Out" <- w2
